vi "subFindAttributeByName.vi"(8 "error in (no error)":errorcluster, 9 "key":string, 11 "Node Reg in":refnum<k20>) -> (0 "error out":errorcluster, 1 "value":string, 2 "key found?":bool, 3 "Node Reg":refnum<k20>)   [LabVIEW 2020, in "DefaultExtensions.lvlib" / "CDefaultRuleFileParser.lvclass"]
uses:
  CDefaultRuleFileParser.lvclass
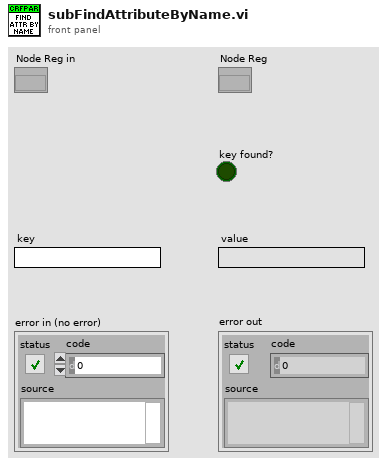
[diagram p1: front panel]
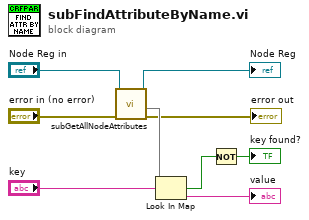
[diagram p0: block diagram]
diagram:
  n1 = call "subGetAllNodeAttributes.vi"("error in (no error)"="error in (no error)", "Node Reg in"="Node Reg in") -> ("error out"=→"error out":errorcluster, "Attributes"=w8:map{string, string}, "Node Reg"=→"Node Reg":refnum<k20>)  [unwired: 7 in]
  n2 = Look In Map(map=w8, key="key") -> (key not found?=w6:bool, value=→"value":string)  [unwired: 1 in]
  n3 = Not(x=w6) -> (.not. x?=→"key found?":bool)
